vi "wformFileWrite.vi"() -> ()   [LabVIEW 2014]
uses:
  <vilib>/Waveform/WDTFileIO.llb/ Write Waveforms to File (1D).vi
  <vilib>/measure/NI_MABase.lvlib
panel:
  out "Saved Waveform Graph":waveform(dbl)[](graph)
  out "Waveform File I/O Error":errorcluster
  in  "Number of Waveforms":i32(slide) scale=0.0..6.0
  out "Waveform file path":path
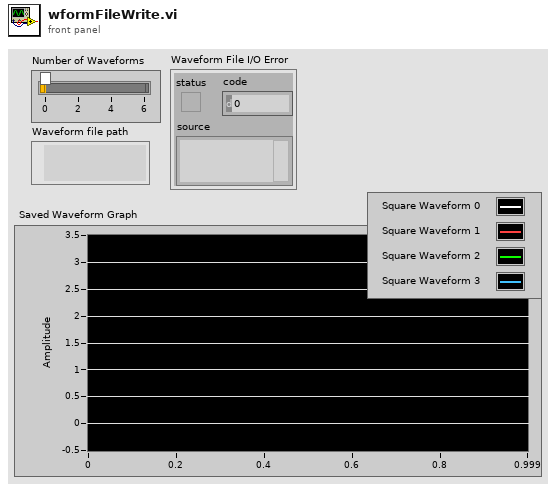
[diagram p1: front panel]
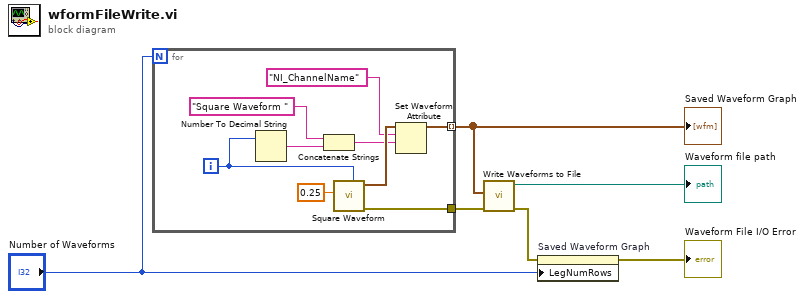
[diagram p0: block diagram]
diagram:
  n1 = for {
    N: "Number of Waveforms" -> [_]
    tunnel: [w15] -> w6
    tunnel: [w13] -> w4 mode=indexing
    i -> [w8]
    n2 = Number To Decimal String(number=w8) -> (decimal integer string=w10:string)  [unwired: 1 in]
    n3 = Concatenate Strings("Square Waveform ", w10) -> (w9:string)
    n4 = call <vilib>:"Square Waveform.vi"("offset"=w8, "amplitude"=0.25) -> ("error out"=w15:errorcluster, "signal out"=w14:waveform(dbl))  [unwired: 8 in]
    n5 = Set Waveform Attribute(5:w9, 6:"NI_ChannelName" ("name"), 7:w14) -> (3:w13:waveform(dbl))  [unwired: 1 in, 2 out]
  }
  "Saved Waveform Graph" <- w4
  n6 = call-poly <vilib>:"Write Waveforms to File.vi"("error in (no error)"=w6, "waveform array"=w4) -> ("error out"=w2:errorcluster, "new file path (Not A Path if cancelled)"=→"Waveform file path":path)  [unwired: 8 in]
  n7 = property on="Saved Waveform Graph" class="WFGraph (strict)"(error in=w2, "LegNumRows"="Number of Waveforms") -> (error out=→"Waveform File I/O Error":errorcluster)  [unwired: 1 in, 1 out]
